vi "Example Graph - DustDensity Callback.vi"(4 "Dust Density":refnum<user-event>, 5 "Event Data":cluster{"sender":refnum<k24>, "dustDensity":i32}, 6 "Control Ref":refnum<k24>, 7 "Event Common Data":T1) -> ()   [LabVIEW 2013]
uses:
  C:/tf/play/labview/Tinkerforge.dll
  Tinkerforge.dll
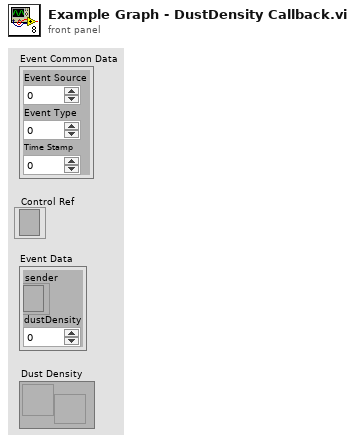
[diagram p1: front panel]
types:
  T1 = cluster{"Event Source":i32, "Event Type":u32, "Time Stamp":u32}
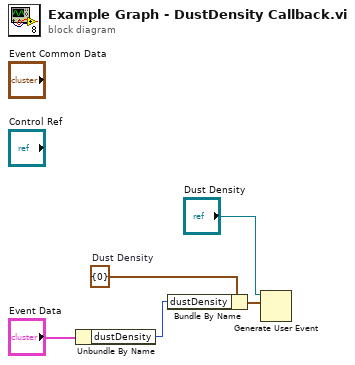
[diagram p0: block diagram]
diagram:
  w4 = cluster{"dustDensity":i32} {"dustDensity"=0}  # Dust Density
  n1 = Unbundle By Name("Event Data") -> ("dustDensity"=w3:i32)
  n2 = Bundle By Name(cluster=w4, "dustDensity"=w3) -> (w2:cluster{"dustDensity":i32})
  n3 = Generate User Event(user event="Dust Density", event data cluster=w2) -> ()  [unwired: 2 in, 2 out]
